vi "SubVI_TogglyBoi2_Teleop.vi"(10 "Boolean in":bool) -> (2 "Boolean out":bool)   [LabVIEW 2017]
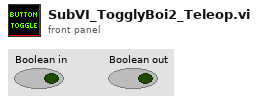
[diagram p1: front panel]
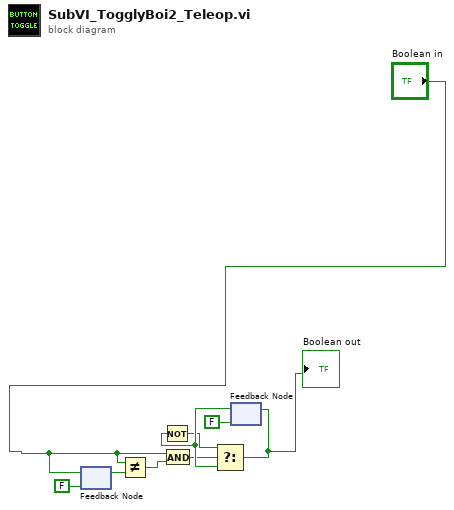
[diagram p0: block diagram]
diagram:
  n1 = feedback #1(FALSE ("Joystick In")) -> (w1:bool)
  n2 = feedback-in #1("Boolean in") -> ()
  n3 = Not Equal?(x="Boolean in", y=w1) -> (x != y?=w2:bool)
  n4 = And(x="Boolean in", y=w2) -> (x .and. y?=w3:bool)
  n5 = feedback #2(FALSE) -> (w5:bool)
  n6 = Not(x=w5) -> (.not. x?=w4:bool)
  n7 = Select(t=w4, s=w3, f=w5) -> (s? t:f=w9:bool)
  "Boolean out" <- w9
  n8 = feedback-in #2(w9) -> ()
